vi "New.vi"(5 "fifo options":T1, 7 "fifo depths (10)":u32=10, 8 "error in (no error)":errorcluster, 11 "Dispatcher Interface type":refnum<class "Dispatcher Interface.lvclass">) -> (0 "error out":errorcluster, 3 "Dispatcher Interface":refnum<class "Dispatcher Interface.lvclass">)   [LabVIEW 2021, in "DSF Core.lvlib" / "Dispatcher Interface.lvclass"]
uses:
  Dispatcher Interface.lvclass
  C:/dev/git/custom-devices/niveristand-data-sharing-framework-custom-device/Source/Core/Classes/Interface/Interface.lvclass
  Typedefs/DSF FIFO Options.ctl
  Response Data.ctl
  Response.ctl
  Parameters.ctl
  Command Data.ctl
  Command.ctl
  FIFO Descriptors.ctl
  FIFO Descriptor.ctl
  Interface.lvclass/Interface.ctl
  Create RT FIFO.vi
  Interface.lvclass
  Framework/Framework.lvclass
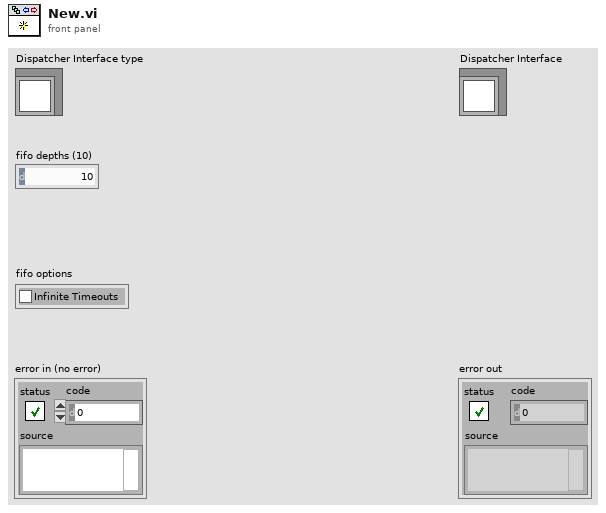
[diagram p1: front panel]
types:
  T1 = typedef "DSF Core.lvlib/Framework.lvclass/DSF FIFO Options.ctl" = cluster{"Infinite Timeouts":bool}
  T2 = typedef "DSF Core.lvlib/Dispatcher Interface.lvclass/Response Data.ctl" = cluster{"Response":T3, "Parameters":T4}
  T3 = typedef "DSF Core.lvlib/Dispatcher Interface.lvclass/Response.ctl" = enum8{"General Ack", "Error", "Shutting Down"}
  T4 = typedef "DSF Core.lvlib/Dispatcher Interface.lvclass/Parameters.ctl" = cluster{"arg1":u64, "arg2":u64}
  T5 = typedef "DSF Core.lvlib/Dispatcher Interface.lvclass/Command Data.ctl" = cluster{"Command":T6, "Parameters":T4}
  T6 = typedef "DSF Core.lvlib/Dispatcher Interface.lvclass/Command.ctl" = enum8{"Idle", "Start", "Rx", "Tx", "Set Inline Buffer", "Shutdown", "Error"}
  T7 = typedef "DSF Core.lvlib/Interface.lvclass/FIFO Descriptors.ctl" = cluster{"command fifo":T8, "response fifo":T8, "error fifo":T8}
  T8 = typedef "DSF Core.lvlib/Interface.lvclass/FIFO Descriptor.ctl" = cluster{"fifo depth":u32, "element size":u32}
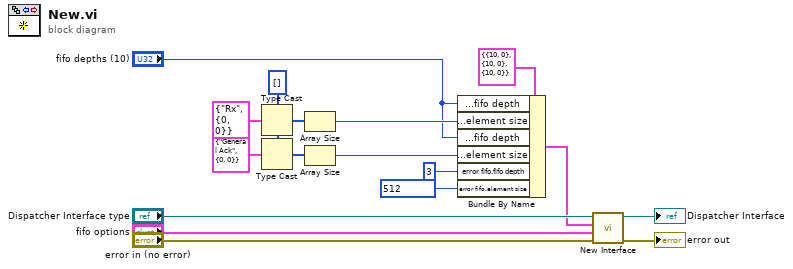
[diagram p0: block diagram]
diagram:
  w4 = u8[] [] ("element")
  n1 = Type Cast(type=w4, x=T5 {"Command"=enum."Rx", "Parameters"={"arg1"=0, "arg2"=0}} ("Dispatcher Command")) -> (*(type *) &x=w10:u8[])
  n2 = Type Cast(type=w4, x=T2 {"Response"=enum."General Ack", "Parameters"={"arg1"=0, "arg2"=0}} ("Dispatcher Response")) -> (*(type *) &x=w8:u8[])
  n3 = Array Size(array=w10) -> (size(s)=w9:i32)
  n4 = Array Size(array=w8) -> (size(s)=w6:i32)
  n5 = Bundle By Name(cluster=T7 {"command fifo"={"fifo depth"=10, "element size"=0}, "response fifo"={"fifo depth"=10, "element size"=0}, "error fifo"={"fifo depth"=10, "element size"=0}} ("fifo descriptors"), "command fifo.fifo depth"="fifo depths (10)", "command fifo.element size"=w9, "response fifo.fifo depth"="fifo depths (10)", "response fifo.element size"=w6, "error fifo.fifo depth"=u32 3, "error fifo.element size"=u32 512 ("element size")) -> (w2:T7)
  n6 = call "New Interface.vi"("error in (no error)"="error in (no error)", "fifo options"="fifo options", "fifo descriptors"=w2, "Interface type"="Dispatcher Interface type") -> ("error out"=→"error out":errorcluster, "Interface"=→"Dispatcher Interface":refnum<class "Dispatcher Interface.lvclass">)  [unwired: 6 in]
